vi "Test Assertion Type for Fail If Equal.vi"(8 "error in (no error)":errorcluster, 11 "Test Assertion Results in":refnum<class "Assertion Result Test.lvclass">) -> (0 "error out":errorcluster, 3 "Test Assertion Results out":refnum<class "Assertion Result Test.lvclass">)   [LabVIEW 2020, in "LUnit Tests.lvlib" / "Assertion Result Test.lvclass"]
uses:
  Assertion Result Test.lvclass
  Test Dummys/Test Case Test Double/Test Case Test Double.lvclass
  source/Framework/Result Types/Assertion Result/Public/TypeDefs/Assertion Type.ctl
  source/Framework/Result Types/Assertion Result/Assertion Result.lvlib
  <vilib>/Astemes/LUnit/Test Case.lvclass
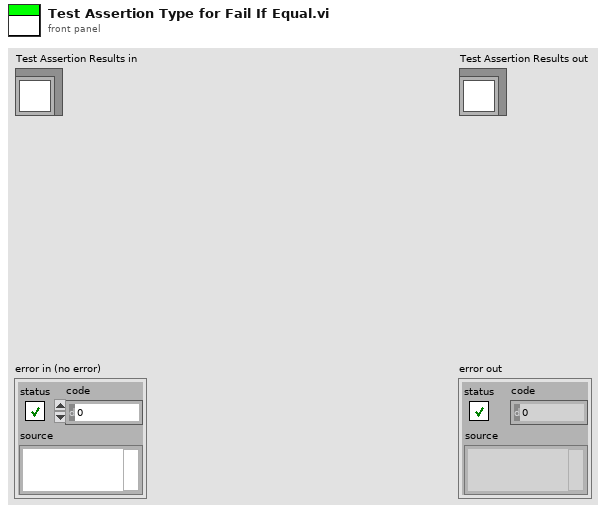
[diagram p1: front panel]
types:
  T1 = typedef "Assertion Result.lvlib/Assertion Type.ctl" = enum16{"None", "Pass", "Fail", "Skip", "Pass if Equal", "Fail if Equal", "Pass if Error", "Fail if Error", "Pass if", "Fail if"}
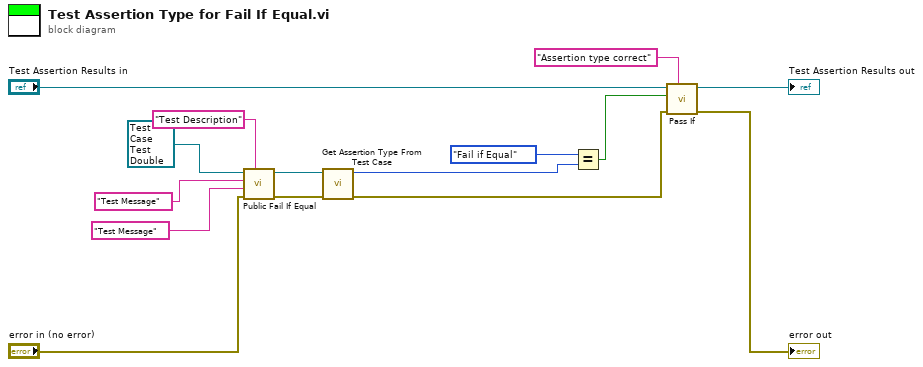
[diagram p0: block diagram]
diagram:
  n1 = call "Public Fail If Equal.vi"("Description"="Test Description", "error in (no error)"="error in (no error)", "Actual"="Test Message" ("Message"), "Expected"="Test Message" ("Message"), "Test Case Test Double in"=refnum<class "Test Case Test Double.lvclass"> refnum ("Test Case Test Double.lvclass")) -> ("error out"=w12:errorcluster, "Test Case Test Double out"=w13:refnum<class "Test Case Test Double.lvclass">)  [unwired: 5 in]
  n2 = call "Get Assertion Type From Test Case.vi"("error in (no error)"=w12, "Test Case Test Double in"=w13) -> ("error out"=w1:errorcluster, "Assertion Type"=w2:T1)  [unwired: 8 in]
  n3 = Equal?(x=Assertion_Type."Fail if Equal" ("Assertion Type"), y=w2) -> (x = y?=w5:bool)
  n4 = call <vilib>:"Pass If.vi"("Description"="Assertion type correct", "error in (no error)"=w1, "Pass?"=w5, "LUnit Test Case In"="Test Assertion Results in") -> ("error out"=→"error out":errorcluster, "LUnit Test Case Out"=→"Test Assertion Results out":refnum<class "Assertion Result Test.lvclass">)  [unwired: 6 in]
